vi "Get Selected Application Instance.vi"(11 "Configuration":T1) -> (3 "Application out":refnum<vi>)   [LabVIEW 2013, in "LVTM.lvlib"]
uses:
  LVTM.lvlib
  Controls_LVTM/LVTM_Config_Info.ctl
  Controls_LVTM/View.ctl
  Controls_LVTM/SharedDataDVR.ctl
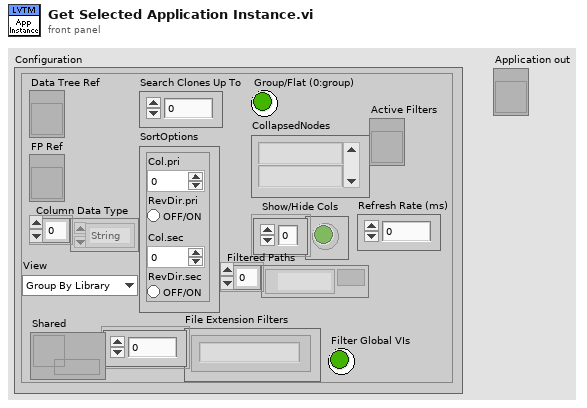
[diagram p1: front panel]
types:
  T1 = typedef "LVTM.lvlib/LVTM_Config_Info.ctl" = cluster{"Data Tree Ref":refnum<vi>, "FP Ref":refnum<vi>, "Column Data Type":enum16{"String", "Numeric"}[], "Search Clones Up To":i32, "SortOptions":cluster{"Col.pri":i32, "RevDir.pri":bool, "Col.sec":i32, "RevDir.sec":bool}, "Group/Flat (0:group)":bool, "CollapsedNodes":string[], "Show/Hide Cols":bool[], "Filtered Paths":path[], "View":T2, "File Extension Filters":string[], "Filter Global VIs":bool, "Shared":refnum<data-value>, "Active Filters":refnum<vi>, "Refresh Rate (ms)":i32}
  T2 = typedef "LVTM.lvlib/View.ctl" = enum16{"Group By Library", "Group By Folder", "Flat List"}
  T3 = typedef "LVTM.lvlib/SharedDataDVR.ctl" = cluster{"App":refnum<vi>, "VIs":string[]}
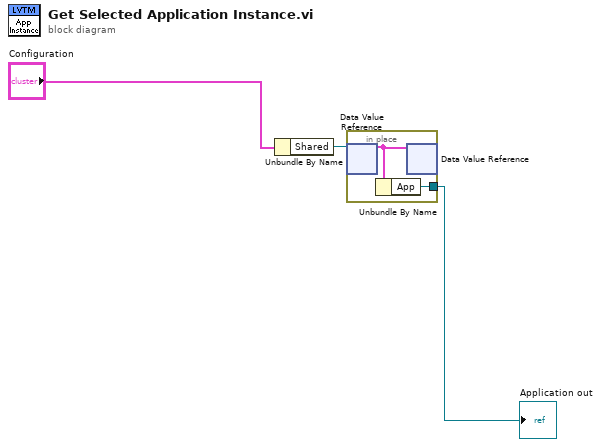
[diagram p0: block diagram]
diagram:
  n1 = Unbundle By Name("Configuration") -> ("Shared"=w1:refnum<data-value>)
  n2 = in-place {
    in-place-border: [w4] -> w3
    n3 = in-place-dvr #1(w1) -> (w5:T3)  [unwired: 1 out]
    n4 = Unbundle By Name(w5) -> ("App"=w4:refnum<vi>)
    n5 = in-place-dvr #1(w5) -> ()  [unwired: 2 out]
  }
  "Application out" <- w3
